vi "To ISO8601 Time.vi"(0 "Time Stamp":timestamp) -> (2 "String":string)   [LabVIEW 2013, in "JUnit XML.lvlib"]
uses:
  JUnit XML.lvlib
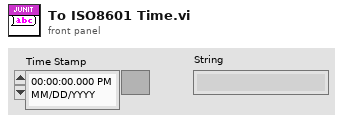
[diagram p1: front panel]
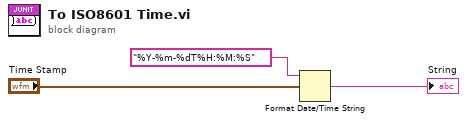
[diagram p0: block diagram]
diagram:
  n1 = Format Date/Time String(time format string (%c)="%Y-%m-%dT%H:%M:%S", seconds (now)="Time Stamp") -> (date/time string=→"String":string)  [unwired: 1 in]
